vi "Create.vi"(8 "error in (no error)":errorcluster) -> (0 "error out":errorcluster, 3 "Framework Performance":refnum<class "Framework Performance.lvclass">)   [LabVIEW 2017, in "DSF Core.lvlib" / "Framework Performance.lvclass"]
uses:
  Framework Performance.lvclass
  <vilib>/NI/Memory Manager/Classes/Pointer/Pointer.lvclass
  Framework Performance.lvclass/Framework Performance.ctl
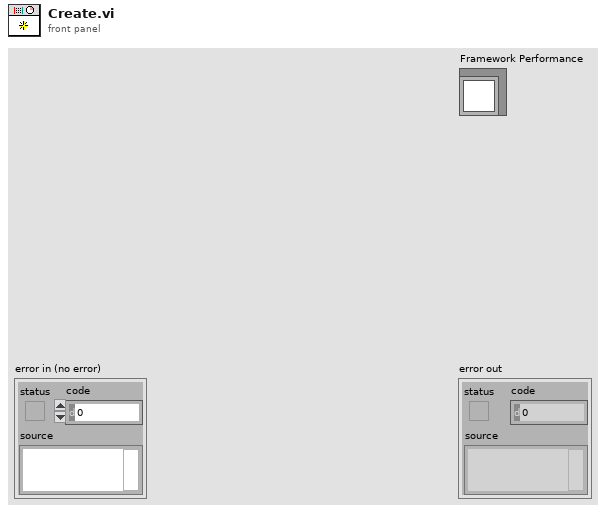
[diagram p1: front panel]
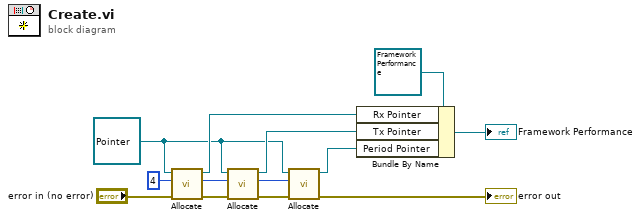
[diagram p0: block diagram]
diagram:
  w1 = refnum<class "Pointer.lvclass"> refnum ("Pointer in")
  w4 = u64 4 ("count (1)")
  n1 = call-dynamic "Allocate.vi"("error in (no error)"="error in (no error)", "size"=w4, "Pointer in"=w1) -> ("error out"=w7:errorcluster, "Pointer out"=w8:refnum<class "Pointer.lvclass">)  [unwired: 7 in]
  n2 = call-dynamic "Allocate.vi"("error in (no error)"=w7, "size"=w4, "Pointer in"=w1) -> ("error out"=w5:errorcluster, "Pointer out"=w6:refnum<class "Pointer.lvclass">)  [unwired: 7 in]
  n3 = call-dynamic "Allocate.vi"("error in (no error)"=w5, "size"=w4, "Pointer in"=w1) -> ("error out"=→"error out":errorcluster, "Pointer out"=w3:refnum<class "Pointer.lvclass">)  [unwired: 7 in]
  n4 = Bundle By Name(cluster=refnum<class "Framework Performance.lvclass"> refnum ("Framework Performance in"), "Rx Pointer"=w8, "Tx Pointer"=w6, "Period Pointer"=w3) -> (→"Framework Performance":refnum<class "Framework Performance.lvclass">)
